vi "set_running_mode.vi"(3 "error in":errorcluster, 4 "Running mode":T1 items=["close_loop", "replay"], 5 "Configuration in":string) -> (0 "error out":errorcluster, 2 "Configuration out":string)   [LabVIEW 2019]
doc: "Builds a string using the simulator configuration and using a running mode chosen by the user."
uses:
  controls/running_mode.ctl
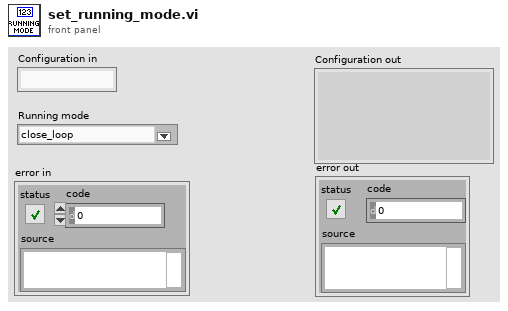
[diagram p1: front panel]
types:
  T1 = typedef "running_mode.ctl" = i32
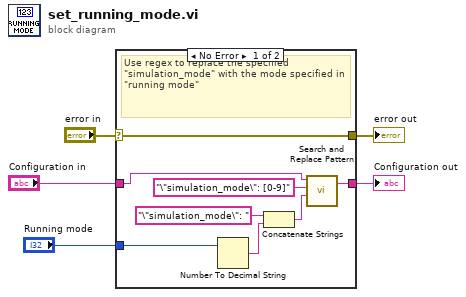
[diagram p0: block diagram]
diagram:
  n1 = case shown="No Error" "error in" {
    selector: "error in" -> [w6 w14]
    tunnel: "Running mode" -> [w8 _]
    tunnel: "Configuration in" -> [w9 w15]
    tunnel: [w7 w15] -> w3
    tunnel: [w6 w14] -> w1
    frame No Error {
      # "Use regex to replace the specified \"simulation_mode\" with the mode specified in \"running mode\""
      n2 = Number To Decimal String(number=w8) -> (decimal integer string=w12:string)  [unwired: 1 in]
      n3 = Concatenate Strings("\"simulation_mode\": " ("regular expression (\"\")"), w12) -> (w13:string)
      n4 = call <vilib>:"Search and Replace Pattern.vi"("string"=w9, "regular expression (\"\")"="\"simulation_mode\": [0-9]" ("regular expression (\"\")"), "replace string (\"\")"=w13) -> ("result string"=w7:string)  [unwired: 2 in, 1 out]
    }
    frame Error {
    }
  }
  "Configuration out" <- w3
  "error out" <- w1
